vi "WPI_CAN_PCMSend.vi"(11 "Pneumatics Control Module (0)":u8) -> (3 "Pneumatics Control Module Out":u8)   [LabVIEW 2017]
uses:
  <vilib>/Rock Robotics/WPI/CAN/PCM/WPI_CAN_PCMMessageIDs.ctl
  <vilib>/Rock Robotics/WPI/CAN/PCM/WPI_CAN_PCMGlobalOps.ctl
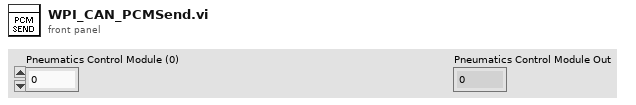
[diagram p1: front panel]
types:
  T1 = typedef "WPI_CAN_PCMGlobalOps.ctl" = enum16{"Read For Send", "Write After Receive", "Set Solenoids", "Set Closed Loop", "Clear Sticky Faults", "Get All", "Write Error", "Write After Receive Blacklist", "Set Control Frame Rate"}
  T2 = cluster{"Solenoid Status":bool[], "Battery Voltage":dbl, "Solenoid Voltage":dbl, "Compressor Current":dbl, "Pneumatic / Fault Systems":cluster{"CompressorEnabled":bool, "StickySolenoidFault":bool, "StickyCompressorFault":bool, "SolenoidFault":bool, "CompressorFault":bool, "HardwareFault":bool, "ClosedLoopStatus":bool, "PressureStatus":bool}, "Module Enabled":bool, "ClosedLoopSuggestedOutput":bool, "CAN Error":errorcluster, "Sticky Solenoid Faults":bool[]}
  T3 = typedef "WPI_CAN_PCMMessageIDs.ctl" = u32
  T4 = cluster{"Solenoids":bool[], "Closed Loop Enable":bool, "Clear Sticky Faults":bool, "Control Frame Rate Ms":i32}
  T5 = cluster{"Solenoid Status":bool[], "Battery Voltage":dbl, "Solenoid Voltage":dbl, "Compressor Current":dbl, "CompressorEnabled":bool, "StickySolenoidFault":bool, "StickyCompressorFault":bool, "SolenoidFault":bool, "CompressorFault":bool, "HardwareFault":bool, "ClosedLoopStatus":bool, "PressureStatus":bool, "Module Enabled":bool, "ClosedLoopSuggestedOutput":bool, "CAN Error":errorcluster, "Sticky Solenoid Faults":bool[]}
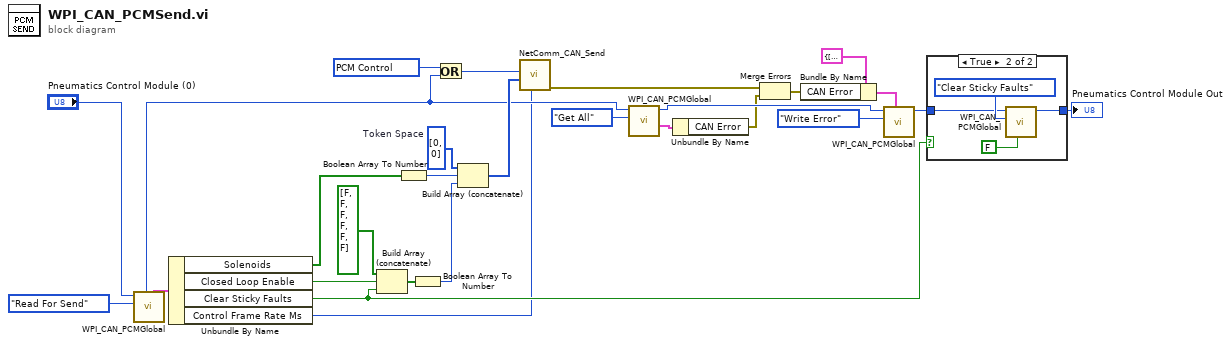
[diagram p0: block diagram]
diagram:
  w23 = u8[] [0, 0]  # Token Space
  w21 = T3 151264256 items=["PCM Control"=151264256, "PCM Status"=151262208, "PCM Status Fault"=151262272, "PCM Debug"=151262336]
  n1 = call <vilib>:"WPI_CAN_PCMGlobal.vi"("Operation"=WPI_CAN_PCMGlobalOps."Read For Send", "Pneumatics Control Module (0)"="Pneumatics Control Module (0)") -> ("Pneumatics Control Module Out"=w5:u8, "Read For Send"=w18:T4)  [unwired: 7 in, 1 out]
  n2 = Unbundle By Name(w18) -> ("Solenoids"=w16:bool[], "Closed Loop Enable"=w17:bool, "Clear Sticky Faults"=w2:bool, "Control Frame Rate Ms"=w1:i32)
  n3 = Build Array (concatenate)(bool[] [FALSE, FALSE, FALSE, FALSE, FALSE, FALSE] ("Data"), w17, w2) -> (w26:bool[])
  n4 = Boolean Array To Number(Boolean array=w16) -> (number=w22:u8)
  n5 = Boolean Array To Number(Boolean array=w26) -> (number=w27:u8)
  n6 = Or(x=w21, y=w5) -> (x .or. y?=w20:T3)
  n7 = Build Array (concatenate)(w23, w22, w27) -> (w24:u8[])
  n8 = call <vilib>:"NetComm_CAN_Send.vi"("Period (ms)"=w1, "Data"=w24, "Message ID"=w20) -> ("error out"=w9:errorcluster)  [unwired: 8 in]
  n9 = call <vilib>:"WPI_CAN_PCMGlobal.vi"("Operation"=WPI_CAN_PCMGlobalOps."Get All", "Pneumatics Control Module (0)"=w5) -> ("Get All"=w10:T5, "Pneumatics Control Module Out"=w11:u8)  [unwired: 7 in, 1 out]
  n10 = Unbundle By Name(w10) -> ("CAN Error"=w8:errorcluster)
  n11 = Merge Errors(w9, w8) -> (w7:errorcluster)
  n12 = Bundle By Name(cluster=T2 {"Solenoid Status"=[], "Battery Voltage"=0.0, "Solenoid Voltage"=0.0, "Compressor Current"=0.0, "Pneumatic / Fault Systems"={"CompressorEnabled"=FALSE, "StickySolenoidFault"=FALSE, "StickyCompressorFault"=FALSE, "SolenoidFault"=FALSE, "CompressorFault"=FALSE, "HardwareFault"=FALSE, "ClosedLoopStatus"=FALSE, "PressureStatus"=FALSE}, "Module Enabled"=FALSE, "ClosedLoopSuggestedOutput"=FALSE, "CAN Error"={"status"=FALSE, "code"=0, "source"=""}, "Sticky Solenoid Faults"=[]} ("Write After Receive"), "CAN Error"=w7) -> (w13:T2)
  n13 = call <vilib>:"WPI_CAN_PCMGlobal.vi"("Write After Receive"=w13, "Operation"=WPI_CAN_PCMGlobalOps."Write Error", "Pneumatics Control Module (0)"=w11) -> ("Pneumatics Control Module Out"=w4:u8)  [unwired: 6 in, 2 out]
  n14 = case shown="True" w2 {
    tunnel: w4 -> [w28 w31]
    tunnel: [w28 w30] -> w3
    frame False {
    }
    frame True {
      n15 = call <vilib>:"WPI_CAN_PCMGlobal.vi"("Set Value"=FALSE, "Operation"=WPI_CAN_PCMGlobalOps."Clear Sticky Faults", "Pneumatics Control Module (0)"=w31) -> ("Pneumatics Control Module Out"=w30:u8)  [unwired: 6 in, 2 out]
    }
  }
  "Pneumatics Control Module Out" <- w3
